vi "실습 2-4, Velocity 제어.vi"() -> ()   [LabVIEW 2014]
uses:
  <vilib>/Motion/FlexMotion/CustomControls/CustomControls.llb/AxisOrVectorSpace To Configure.flx
  <vilib>/Motion/FlexMotion/FunctionsVIs/StartStopMotion.llb/Start Motion (8 axes).flx
  <vilib>/Motion/FlexMotion/FunctionsVIs/StartStopMotion.llb/Stop Motion (8 axes).flx
panel:
  in  "정지":bool
  in  "Velocity (10000)":i32(slide)=1480 scale=-36000.0..36000.0
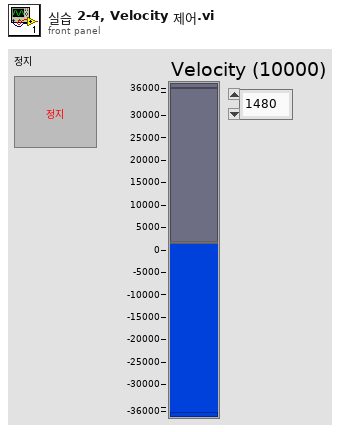
[diagram p1: front panel]
types:
  T1 = enum16{"Absolute Position", "Relative Position", "Velocity", "Relative to Cap Pos", "Modulus Position", "Absolute Contouring", "Relative Contouring"}
  T2 = typedef "AxisOrVectorSpace To Configure.flx" = u16
  T3 = typedef "Resource Out (Enum).flx" = u16
  T4 = typedef "Bd Id Out" = u8
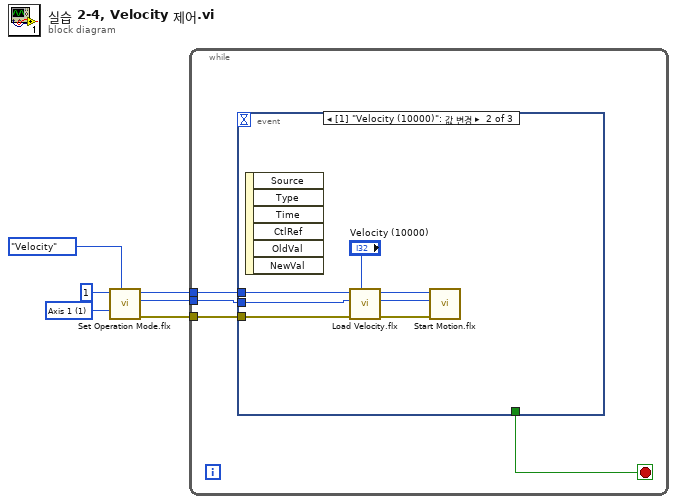
[diagram p0: block diagram]
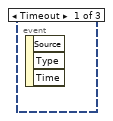
[diagram p2: hidden frame]
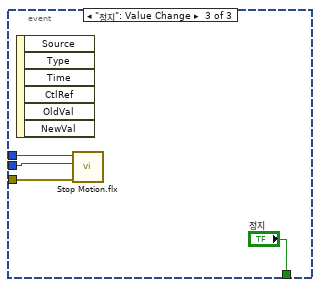
[diagram p3: hidden frame]
diagram:
  w5 = T2 1 items=["Axis 1"=1, "Axis 2"=2, "Axis 3"=3, "Axis 4"=4, "Axis 5"=5, "Axis 6"=6, "Axis 7"=7, "Axis 8"=8, "Vector Space 1"=17, "Vector Space 2"=18, "Vector Space 3"=19, "Vector Space 4"=20] ("Axis or Vector Space")
  n1 = call <vilib>:"Set Operation Mode.flx"("Position Mode (Absolute)"=T1."Velocity", "Axis or Vector Space"=w5, "Board ID"=u8 1) -> ("error out"=w1:errorcluster, "Resource Output"=w2:T3, "Bd ID Out"=w3:T4)  [unwired: 3 in]
  n2 = while {
    tunnel: w3 -> [w10]
    tunnel: w2 -> [w9]
    tunnel: w1 -> [w8]
    stop <- w7 stop-if-true
    n3 = event shown="[1] \"Velocity (10000)\": 값 변경" {
      selector: _ -> [_ _ _]
      dyn-events: _ -> [_ _ _]
      timeout: _ -> [_ _ _]
      tunnel: w10 -> [_ w16 w21]
      tunnel: w9 -> [_ w15 w20]
      tunnel: w8 -> [_ w14 w19]
      tunnel: [_ _ "정지"] -> w7
      event Timeout {
        n4 = event-data() -> ()  [unwired: 1 in, 3 out]
      }
      event "Velocity (10000)": Value Change {
        n5 = event-data() -> ()  [unwired: 1 in, 6 out]
        n6 = call <vilib>:"Load Velocity.flx"("Velocity (10000)"="Velocity (10000)", "error in (no error)"=w14, "Axis or Vector Space"=w15, "Board ID"=w16) -> ("error out"=w11:errorcluster, "Resource Output"=w12:T3, "Bd ID Out"=w13:T4)  [unwired: 3 in]
        n7 = call-poly <vilib>:"Start Motion.flx"("error in (no error)"=w11, "Axis or Vector Space"=w12, "Board ID"=w13) -> ()  [unwired: 3 in, 3 out]
      }
      event "정지": Value Change {
        n8 = event-data() -> ()  [unwired: 1 in, 6 out]
        n9 = call-poly <vilib>:"Stop Motion.flx"("error in (no error)"=w19, "Axis or Vector Space"=w20, "Board ID"=w21) -> ()  [unwired: 4 in, 3 out]
      }
    }
  }
